vi "create_project.vi"(11 "设置输入":T1 {"串口通信UI"."Format" items=["标准帧", "扩展帧"]; "串口通信UI"."Type" items=["数据帧", "远程帧"]; "串口通信UI"."ID" format="0x%x"; "串口通信UI"."Fliter" items=["接收所有类型"=1, "只接收标准帧"=2, "只接收扩展帧"=3]; "串口通信UI"."kBaudRate" items=["5k bps"=1, "10k bps"=2, "20k bps"=3, "40k bps"=4, "50k bps"=5, "80k bps"=6, "100k bps"=7, "125k bps"=8, "200k bps"=9, "250k bps"=10, "400k bps"=11, "500k bps"=12, "666k bps"=13, "800k bps"=14, "1000k bps"=15, "33.33k bps"=16, "66.66k bps"=17, "83.33k bps"=18]; "串口通信UI"."Mode" items=["正常工作", "仅侦听模式", "自测模式（环回）"]; "串口通信UI"."InitFlag" items=["使用界面设置参数"=1]; "串口通信UI"."AccMask" format="%08x"; "串口通信UI"."AccCode" format="%08x"; "串口通信UI"."Channel" items=["通道1", "通道2"]; "串口通信UI"."DevType" items=["USB-CAN"=3, "USB-CAN2"=4]; "安全报警UI"."操作 8" items=["产生报警信息（不发声），等待手动操作", "产生报警信息（发声），等待手动操作", "产生报警信息（不发声），自动刹车", "产生报警信息（发声），自动刹车", "产生报警信息（不发声），立即自动断电，开启泄放电阻", "产生报警信息（发声），立即自动断电，开启泄放电阻"]; "安全报警UI"."操作 7" items=["产生报警信息（不发声），等待手动操作", "产生报警信息（发声），等待手动操作", "产生报警信息（不发声），自动刹车", "产生报警信息（发声），自动刹车", "产生报警信息（不发声），立即自动断电，开启泄放电阻", "产生报警信息（发声），立即自动断电，开启泄放电阻"]; "安全报警UI"."操作 6" items=["产生报警信息（不发声），等待手动操作", "产生报警信息（发声），等待手动操作", "产生报警信息（不发声），自动刹车", "产生报警信息（发声），自动刹车", "产生报警信息（不发声），立即自动断电，开启泄放电阻", "产生报警信息（发声），立即自动断电，开启泄放电阻"]; "安全报警UI"."操作 5" items=["产生报警信息（不发声），等待手动操作", "产生报警信息（发声），等待手动操作", "产生报警信息（不发声），自动刹车", "产生报警信息（发声），自动刹车", "产生报警信息（不发声），立即自动断电，开启泄放电阻", "产生报警信息（发声），立即自动断电，开启泄放电阻"]; "安全报警UI"."操作 4" items=["产生报警信息（不发声），等待手动操作", "产生报警信息（发声），等待手动操作", "产生报警信息（不发声），自动刹车", "产生报警信息（发声），自动刹车", "产生报警信息（不发声），立即自动断电，开启泄放电阻", "产生报警信息（发声），立即自动断电，开启泄放电阻"]; "安全报警UI"."操作 3" items=["产生报警信息（不发声），等待手动操作", "产生报警信息（发声），等待手动操作", "产生报警信息（不发声），自动刹车", "产生报警信息（发声），自动刹车", "产生报警信息（不发声），立即自动断电，开启泄放电阻", "产生报警信息（发声），立即自动断电，开启泄放电阻"]; "安全报警UI"."操作 2" items=["产生报警信息（不发声），等待手动操作", "产生报警信息（发声），等待手动操作", "产生报警信息（不发声），自动刹车", "产生报警信息（发声），自动刹车", "产生报警信息（不发声），立即自动断电，开启泄放电阻", "产生报警信息（发声），立即自动断电，开启泄放电阻"]; "安全报警UI"."操作" items=["产生报警信息（不发声），等待手动操作", "产生报警信息（发声），等待手动操作", "产生报警信息（不发声），自动刹车", "产生报警信息（发声），自动刹车", "产生报警信息（不发声），立即自动断电，开启泄放电阻", "产生报警信息（发声），立即自动断电，开启泄放电阻"]; "串口通信配置"."DevType" items=["USB-CAN"=3, "USB-CAN2"=4]; "串口通信配置"."CanIndex" items=["通道1", "通道2"]; "串口通信配置"."VCI_INIT_CONFIG"."Fliter" items=["接收所有类型"=3, "只接收标准帧"=4, "只接收扩展帧"=7]; "串口通信配置"."VCI_INIT_CONFIG"."Mode" items=["正常工作", "自测模式（环回）", "仅侦听模式"]; "串口通信配置"."VCI_INIT_CONFIG"."InitFlag" items=["使用Flash参数", "使用界面设置参数"]}) -> (3 "设置输出":T1 {"串口通信UI"."Format" items=["标准帧", "扩展帧"]; "串口通信UI"."Type" items=["数据帧", "远程帧"]; "串口通信UI"."ID" format="0x%x"; "串口通信UI"."Fliter" items=["接收所有类型"=1, "只接收标准帧"=2, "只接收扩展帧"=3]; "串口通信UI"."kBaudRate" items=["5k bps"=1, "10k bps"=2, "20k bps"=3, "40k bps"=4, "50k bps"=5, "80k bps"=6, "100k bps"=7, "125k bps"=8, "200k bps"=9, "250k bps"=10, "400k bps"=11, "500k bps"=12, "666k bps"=13, "800k bps"=14, "1000k bps"=15, "33.33k bps"=16, "66.66k bps"=17, "83.33k bps"=18]; "串口通信UI"."Mode" items=["正常工作", "仅侦听模式", "自测模式（环回）"]; "串口通信UI"."InitFlag" items=["使用界面设置参数"=1]; "串口通信UI"."AccMask" format="%08x"; "串口通信UI"."AccCode" format="%08x"; "串口通信UI"."Channel" items=["通道1", "通道2"]; "串口通信UI"."DevType" items=["USB-CAN"=3, "USB-CAN2"=4]; "安全报警UI"."操作 8" items=["产生报警信息（不发声），等待手动操作", "产生报警信息（发声），等待手动操作", "产生报警信息（不发声），自动刹车", "产生报警信息（发声），自动刹车", "产生报警信息（不发声），立即自动断电，开启泄放电阻", "产生报警信息（发声），立即自动断电，开启泄放电阻"]; "安全报警UI"."操作 7" items=["产生报警信息（不发声），等待手动操作", "产生报警信息（发声），等待手动操作", "产生报警信息（不发声），自动刹车", "产生报警信息（发声），自动刹车", "产生报警信息（不发声），立即自动断电，开启泄放电阻", "产生报警信息（发声），立即自动断电，开启泄放电阻"]; "安全报警UI"."操作 6" items=["产生报警信息（不发声），等待手动操作", "产生报警信息（发声），等待手动操作", "产生报警信息（不发声），自动刹车", "产生报警信息（发声），自动刹车", "产生报警信息（不发声），立即自动断电，开启泄放电阻", "产生报警信息（发声），立即自动断电，开启泄放电阻"]; "安全报警UI"."操作 5" items=["产生报警信息（不发声），等待手动操作", "产生报警信息（发声），等待手动操作", "产生报警信息（不发声），自动刹车", "产生报警信息（发声），自动刹车", "产生报警信息（不发声），立即自动断电，开启泄放电阻", "产生报警信息（发声），立即自动断电，开启泄放电阻"]; "安全报警UI"."操作 4" items=["产生报警信息（不发声），等待手动操作", "产生报警信息（发声），等待手动操作", "产生报警信息（不发声），自动刹车", "产生报警信息（发声），自动刹车", "产生报警信息（不发声），立即自动断电，开启泄放电阻", "产生报警信息（发声），立即自动断电，开启泄放电阻"]; "安全报警UI"."操作 3" items=["产生报警信息（不发声），等待手动操作", "产生报警信息（发声），等待手动操作", "产生报警信息（不发声），自动刹车", "产生报警信息（发声），自动刹车", "产生报警信息（不发声），立即自动断电，开启泄放电阻", "产生报警信息（发声），立即自动断电，开启泄放电阻"]; "安全报警UI"."操作 2" items=["产生报警信息（不发声），等待手动操作", "产生报警信息（发声），等待手动操作", "产生报警信息（不发声），自动刹车", "产生报警信息（发声），自动刹车", "产生报警信息（不发声），立即自动断电，开启泄放电阻", "产生报警信息（发声），立即自动断电，开启泄放电阻"]; "安全报警UI"."操作" items=["产生报警信息（不发声），等待手动操作", "产生报警信息（发声），等待手动操作", "产生报警信息（不发声），自动刹车", "产生报警信息（发声），自动刹车", "产生报警信息（不发声），立即自动断电，开启泄放电阻", "产生报警信息（发声），立即自动断电，开启泄放电阻"]; "串口通信配置"."DevType" items=["USB-CAN"=3, "USB-CAN2"=4]; "串口通信配置"."CanIndex" items=["通道1", "通道2"]; "串口通信配置"."VCI_INIT_CONFIG"."Fliter" items=["接收所有类型"=3, "只接收标准帧"=4, "只接收扩展帧"=7]; "串口通信配置"."VCI_INIT_CONFIG"."Mode" items=["正常工作", "自测模式（环回）", "仅侦听模式"]; "串口通信配置"."VCI_INIT_CONFIG"."InitFlag" items=["使用Flash参数", "使用界面设置参数"]})   [LabVIEW 2018, in "menu.lvlib"]
uses:
  menu.lvlib
  Settings/Settings.ctl
  Acquisition/Hardware Configuration.ctl
  Acquisition/Signal Type.ctl
  canstatus.ctl
  <vilib>/Utility/xml.llb/Write to XML File(string).vi
  create_project_Dialog.vi
  Acquisition/Acquisition.lvlib
  Settings/Settings.lvlib
  UI.lvlib
panel:
  in  "error in (no error)":cluster{"状态":bool, "代码":i32, "源":string} caption="错误输入（无错误）"
  out "error out":cluster{"状态":bool, "代码":i32, "源":string} caption="错误输出"
  # "参数配置文件"
  # "输入数据文件"
  # "EHA电机"
  # "模拟电机"
  # "注：每次运行实验时销毁现有所有图像"
  # "参数配置文件"
  # "输入数据文件"
  # "EHA电机"
  # "模拟电机"
  # "注：每次运行实验时销毁现有所有图像"
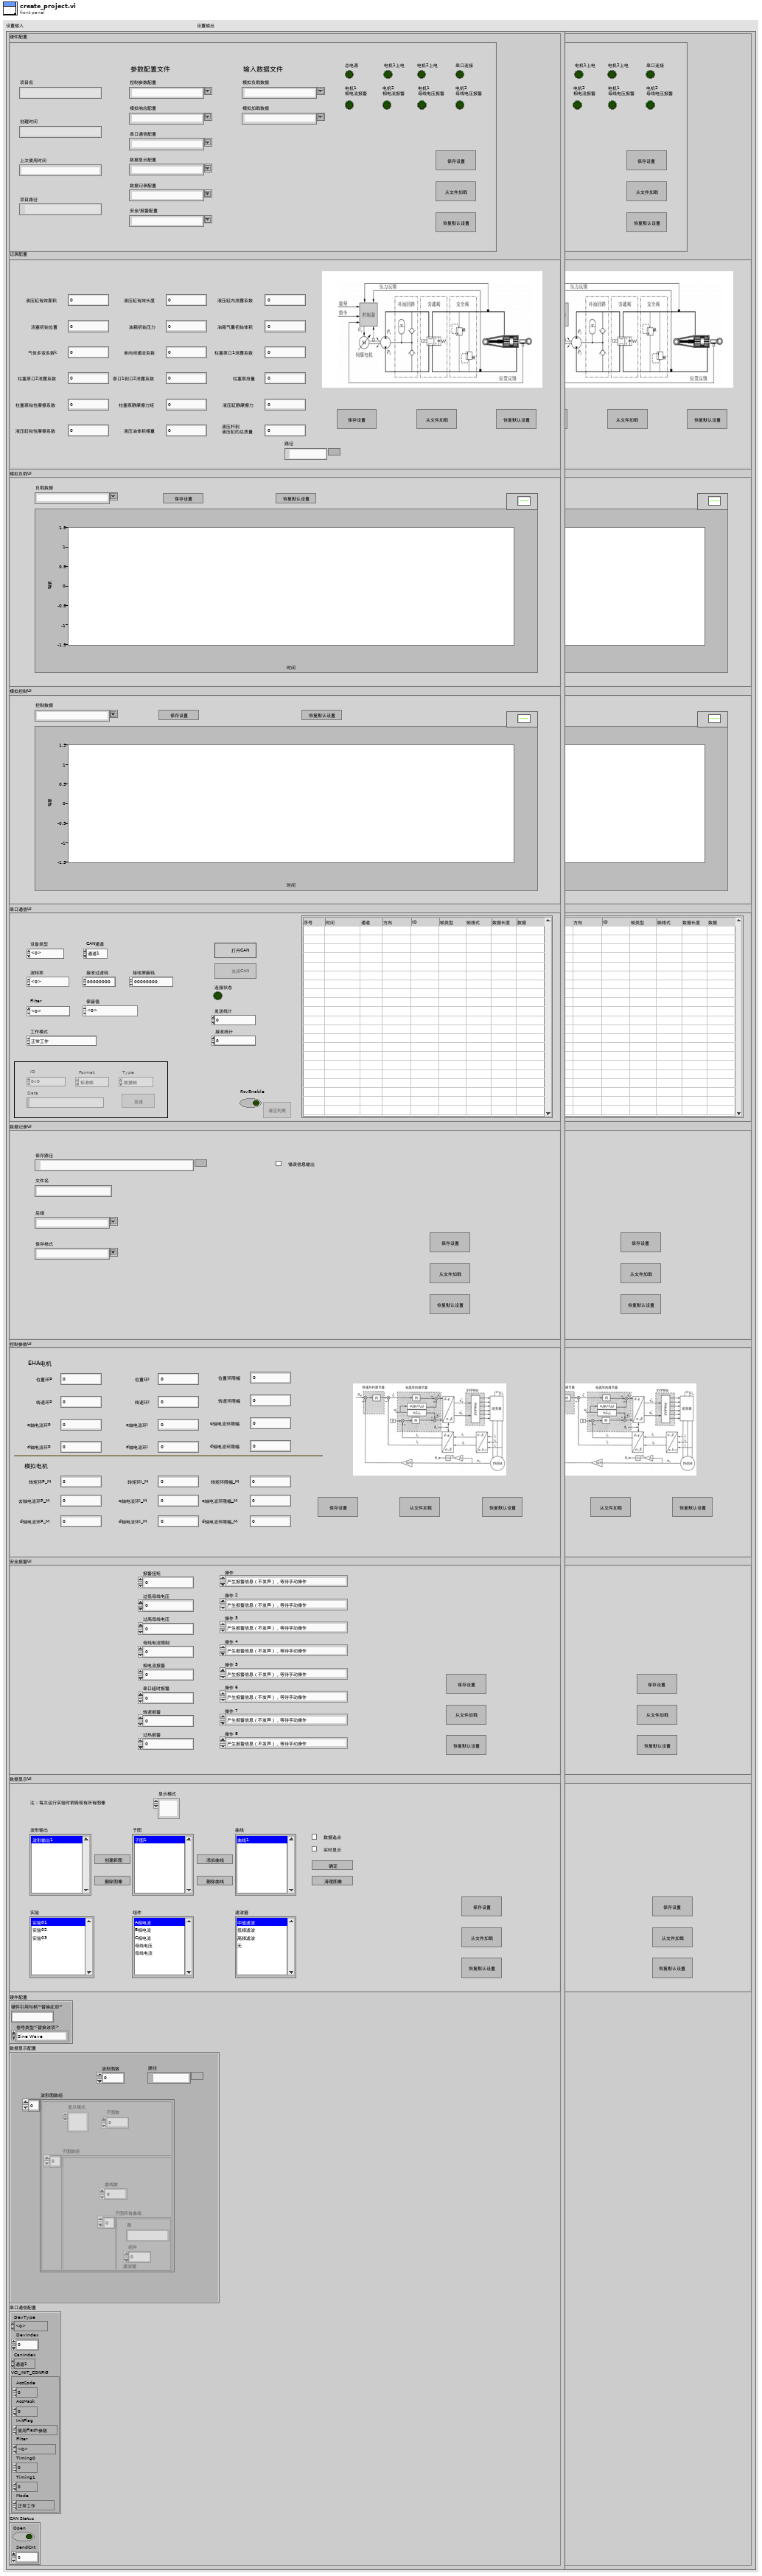
[diagram p1: front panel]
types:
  T1 = typedef "Settings.lvlib/Settings.ctl" = cluster{"当前项目UI":T2, "EHA模拟UI":T3, "模拟负载UI":T4, "模拟控制UI":T5, "串口通信UI":T6, "数据记录UI":T12, "控制参数UI":T13, "安全报警UI":T14, "数据显示UI":T15, "硬件配置":T16, "数据显示配置":T18, "串口通信配置":T22, "CAN Status":T24}
  T2 = typedef "控件 5.ctl" = cluster{"控制参数配置":string, "模拟响应配置":string, "串口通信配置":string, "数据显示配置":string, "数据记录配置":string, "安全/报警配置":string, "模拟负载数据":string, "模拟加载数据":string, "总电源":bool, "电机1上电":bool, "电机2上电":bool, "串口连接":bool, "电机1\n相电流报警":bool, "电机2\n相电流报警":bool, "电机1\n母线电压报警":bool, "电机2\n母线电压报警":bool, "保存设置":bool, "从文件加载":bool, "恢复默认设置":bool, "路径":path, "项目路径":path, "项目名":string, "创建时间":string, "上次使用时间":string}
  T3 = typedef "EHA模拟UI.ctl" = cluster{"液压缸有效面积":dbl, "活塞初始位置":dbl, "气体多变系数k":dbl, "柱塞泵口2泄露系数":dbl, "柱塞泵粘性摩擦系数":dbl, "液压缸粘性摩擦系数":dbl, "液压缸有效长度":dbl, "油箱初始压力":dbl, "单向阀通流系数":dbl, "泵口1到口2泄露系数":dbl, "柱塞泵静摩擦力矩":dbl, "液压油体积模量":dbl, "保存设置":bool, "从文件加载":bool, "恢复默认设置":bool, "路径":path, "液压缸内泄露系数":dbl, "油箱气囊初始体积":dbl, "柱塞泵口1泄露系数":dbl, "柱塞泵排量":dbl, "液压缸静摩擦力":dbl, "液压杆到\n液压缸的总质量":dbl}
  T4 = typedef "控件 9.ctl" = cluster{"负载数据":string, "负载数据 2":waveform(dbl)[], "保存设置":bool, "恢复默认设置":bool}
  T5 = typedef "控件 7.ctl" = cluster{"控制数据":string, "负载数据 2":waveform(dbl)[], "保存设置":bool, "恢复默认设置":bool}
  T6 = typedef "控件 6.ctl" = cluster{"DevType":T7, "Channel":T8, "AccCode":u32, "AccMask":u32, "InitFlag":T9, "Mode":T10, "kBaudRate":u8, "Fliter":T11, "Open":bool, "Close":bool, "连接状态":bool, "SendCnt":u32, "RecvCnt":u32, "Send":bool, "ID":u32, "Data":string, "Type":u8, "Format":u8, "Clear":bool, "list":i32, "路径":path, "RcvEnable":bool}
  T7 = typedef "can库.lvlib/ControlCAN.lvlib/DevType.ctl" = u32
  T8 = typedef "can库.lvlib/ControlCAN.lvlib/CAN Channel.ctl" = u32
  T9 = typedef "can库.lvlib/ControlCAN.lvlib/InitFlag.ctl" = u32
  T10 = typedef "can库.lvlib/ControlCAN.lvlib/Mode.ctl" = u8
  T11 = typedef "can库.lvlib/ControlCAN.lvlib/Fliter.ctl" = u8
  T12 = typedef "控件 3.ctl" = cluster{"保存路径":path, "文件名":string, "后缀":string, "保存格式":string, "复选框":bool, "保存设置":bool, "从文件加载":bool, "恢复默认设置":bool, "路径":path, "TDMS文件引用":refnum<k34>}
  T13 = typedef "控件 1.ctl" = cluster{"d轴电流环P_M":dbl, "转速环P":dbl, "q轴电流环P":dbl, "d轴电流环P":dbl, "转矩环P_M":dbl, "去轴电流环P_M":dbl, "转速环I":dbl, "q轴电流环I":dbl, "d轴电流环I":dbl, "转矩环I_M":dbl, "q轴电流环I_M":dbl, "d轴电流环I_M":dbl, "保存设置":bool, "从文件加载":bool, "恢复默认设置":bool, "路径":path, "位置环P":dbl, "位置环I":dbl, "转速环限幅":dbl, "q轴电流环限幅":dbl, "d轴电流环限幅":dbl, "位置环限幅":dbl, "转矩环限幅_M":dbl, "q轴电流环限幅_M":dbl, "d轴电流环限幅_M":dbl}
  T14 = typedef "控件 4.ctl" = cluster{"报警扭矩":dbl, "过低母线电压":dbl, "过高母线电压":dbl, "母线电流限制":dbl, "相电流报警":dbl, "串口超时报警":dbl, "转速报警":dbl, "过热报警":dbl, "操作":u16, "操作 2":u16, "操作 3":u16, "操作 4":u16, "操作 5":u16, "操作 6":u16, "操作 7":u16, "操作 8":u16, "保存设置":bool, "从文件加载":bool, "恢复默认设置":bool, "路径":path}
  T15 = typedef "控件 2.ctl" = cluster{"保存设置":bool, "从文件加载":bool, "恢复默认设置":bool, "实验":i32, "波形输出":i32, "组件":i32, "曲线":i32, "滤波器":i32, "删除曲线":bool, "清理图像":bool, "添加曲线":bool, "数据选点":bool, "确定按钮":bool, "实时显示":bool, "子图":i32, "显示模式":u16, "路径":path, "删除图像":bool, "创建新图":bool}
  T16 = typedef "Acquisition.lvlib/Hardware Configuration.ctl" = cluster{"硬件引用句柄<替换此项>":string, "信号类型<替换该项>":T17}
  T17 = typedef "Acquisition.lvlib/Signal Type.ctl" = enum16{"Sine Wave", "Square with Noise"}
  T18 = typedef "波形图簇.ctl" = cluster{"波形图数":u32, "波形图数组":T19[], "路径":path}
  T19 = typedef "波形图.ctl" = cluster{"显示模式":u16, "子图数":u32, "子图数组":T20[]}
  T20 = typedef "子图.ctl" = cluster{"子图所有曲线":T21[], "曲线数":u32}
  T21 = typedef "曲线簇.ctl" = cluster{"源":string, "组件":u32, "滤波器":u32}
  T22 = typedef "UI.lvlib/串口通信配置.ctl" = cluster{"DevType":T7, "DevIndex":u32, "CanIndex":T8, "VCI_INIT_CONFIG":T23}
  T23 = typedef "can库.lvlib/ControlCAN.lvlib/VCI_INIT_CONFIG.ctl" = cluster{"AccCode":u32, "AccMask":u32, "InitFlag":T9, "Fliter":T11, "Timing0":u8, "Timing1":u8, "Mode":T10}
  T24 = typedef "UI.lvlib/canstatus.ctl" = cluster{"Open":bool, "SendCnt":u32}
  T25 = cluster{"控制参数配置":string, "模拟响应配置":string, "串口通信配置":string, "数据显示配置":string, "数据记录配置":string, "安全/报警配置":string, "模拟负载数据":string, "模拟加载数据":string, "总电源":bool, "电机1上电":bool, "电机2上电":bool, "串口连接":bool, "电机1\n相电流报警":bool, "电机2\n相电流报警":bool, "电机1\n母线电压报警":bool, "电机2\n母线电压报警":bool, "保存设置":bool, "从文件加载":bool, "恢复默认设置":bool, "路径":path, "项目路径":path, "项目名":string, "创建时间":string, "上次使用时间":string}
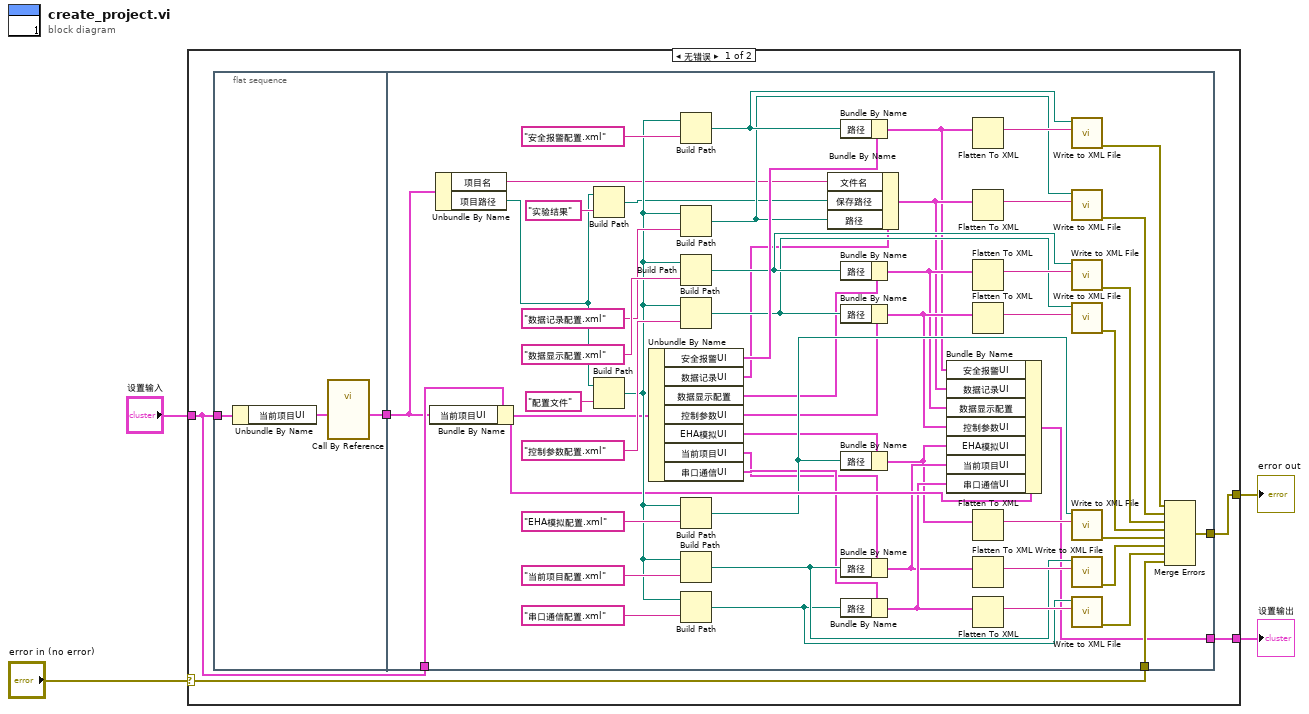
[diagram p0: block diagram]
diagram:
  n1 = case shown="无错误" "error in (no error)" {
    selector: "error in (no error)" -> [w8 w68]
    tunnel: [w7 w68] -> w1
    tunnel: [w9 w67] -> w4
    tunnel: "设置输入" -> [w6 w67]
    frame No Error {
      n2 = flat-sequence {
        tunnel: w6 -> [w11]
        tunnel: [w10] -> w5
        tunnel: [w17] -> w9
        tunnel: w8 -> [w59]
        tunnel: [w51] -> w7
        tunnel: w6 -> [w50]
        tunnel: w5 -> [w42]
        frame #0 {
          n3 = Unbundle By Name(w11) -> ("当前项目UI"=w12:T2)
          n4 = call-by-ref "?"("当前项目配置 输入"=w12) -> ("当前项目配置 输出"=w10:T25)  [unwired: 12 in, 2 out]
        }
        frame #1 {
          n5 = Bundle By Name(cluster=w50, "当前项目UI"=w42) -> (w39:T1)
          n6 = Unbundle By Name(w42) -> ("项目名"=w13:string, "项目路径"=w15:path)
          n7 = Build Path(base path=w15, name or relative path="实验结果") -> (appended path=w14:path)
          n8 = Build Path(base path=w15, name or relative path="配置文件") -> (appended path=w41:path)
          n9 = Unbundle By Name(w39) -> ("安全报警UI"=w38:T14, "数据记录UI"=w25:T12, "数据显示配置"=w27:T18, "控制参数UI"=w26:T13, "EHA模拟UI"=w28:T3, "当前项目UI"=w29:T2, "串口通信UI"=w30:T6)
          n10 = Build Path(base path=w41, name or relative path="安全报警配置.xml") -> (appended path=w37:path)
          n11 = Build Path(base path=w41, name or relative path="数据记录配置.xml") -> (appended path=w36:path)
          n12 = Build Path(base path=w41, name or relative path="数据显示配置.xml") -> (appended path=w35:path)
          n13 = Build Path(base path=w41, name or relative path="控制参数配置.xml") -> (appended path=w34:path)
          n14 = Build Path(base path=w41, name or relative path="EHA模拟配置.xml") -> (appended path=w33:path)
          n15 = Build Path(base path=w41, name or relative path="当前项目配置.xml") -> (appended path=w32:path)
          n16 = Build Path(base path=w41, name or relative path="串口通信配置.xml") -> (appended path=w31:path)
          n17 = Bundle By Name(cluster=w25, "文件名"=w13, "保存路径"=w14, "路径"=w36) -> (w20:T12)
          n18 = Bundle By Name(cluster=w38, "路径"=w37) -> (w19:T14)
          n19 = Bundle By Name(cluster=w27, "路径"=w35) -> (w21:T18)
          n20 = Bundle By Name(cluster=w26, "路径"=w34) -> (w22:T13)
          n21 = Bundle By Name(cluster=w28, "路径"=w33) -> (w18:T3)
          n22 = Bundle By Name(cluster=w29, "路径"=w32) -> (w23:T2)
          n23 = Bundle By Name(cluster=w30, "路径"=w31) -> (w24:T6)
          n24 = Bundle By Name(cluster=w39, "安全报警UI"=w19, "数据记录UI"=w20, "数据显示配置"=w21, "控制参数UI"=w22, "EHA模拟UI"=w18, "当前项目UI"=w23, "串口通信UI"=w24) -> (w17:T1)
          n25 = Flatten To XML(anything=w19) -> (xml string=w52:string)
          n26 = Flatten To XML(anything=w20) -> (xml string=w55:string)
          n27 = Flatten To XML(anything=w21) -> (xml string=w53:string)
          n28 = Flatten To XML(anything=w22) -> (xml string=w54:string)
          n29 = Flatten To XML(anything=w18) -> (xml string=w56:string)
          n30 = Flatten To XML(anything=w23) -> (xml string=w57:string)
          n31 = Flatten To XML(anything=w24) -> (xml string=w58:string)
          n32 = call-poly <vilib>:"Write to XML File.vi"("XML Input"=w52, "XML File Path"=w37) -> ("error out"=w60:errorcluster)  [unwired: 7 in, 2 out]
          n33 = call-poly <vilib>:"Write to XML File.vi"("XML Input"=w55, "XML File Path"=w36) -> ("error out"=w61:errorcluster)  [unwired: 7 in, 2 out]
          n34 = call-poly <vilib>:"Write to XML File.vi"("XML Input"=w53, "XML File Path"=w35) -> ("error out"=w62:errorcluster)  [unwired: 7 in, 2 out]
          n35 = call-poly <vilib>:"Write to XML File.vi"("XML Input"=w54, "XML File Path"=w34) -> ("error out"=w63:errorcluster)  [unwired: 7 in, 2 out]
          n36 = call-poly <vilib>:"Write to XML File.vi"("XML Input"=w56, "XML File Path"=w33) -> ("error out"=w64:errorcluster)  [unwired: 7 in, 2 out]
          n37 = call-poly <vilib>:"Write to XML File.vi"("XML Input"=w57, "XML File Path"=w32) -> ("error out"=w65:errorcluster)  [unwired: 7 in, 2 out]
          n38 = call-poly <vilib>:"Write to XML File.vi"("XML Input"=w58, "XML File Path"=w31) -> ("error out"=w66:errorcluster)  [unwired: 7 in, 2 out]
          n39 = Merge Errors(w60, w61, w62, w63, w64, w65, w66, w59) -> (w51:errorcluster)
        }
      }
    }
    frame Error {
    }
  }
  "error out" <- w1
  "设置输出" <- w4
